vi "Constructor.vi"(10 "Beverage":refnum<class "Beverage.lvclass">, 11 "Milk in":refnum<class "Milk.lvclass">) -> (3 "Milk out":refnum<class "Milk.lvclass">)   [LabVIEW 2011, in "Milk.lvclass"]
uses:
  Milk.lvclass
  Beverage/Beverage.lvclass
  Milk.lvclass/Milk.ctl
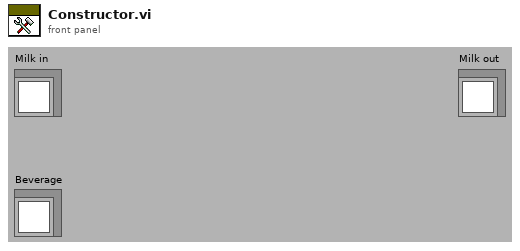
[diagram p1: front panel]
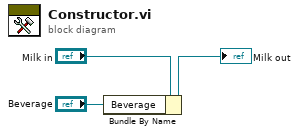
[diagram p0: block diagram]
diagram:
  n1 = Bundle By Name(cluster="Milk in", "Beverage"="Beverage") -> (→"Milk out":refnum<class "Milk.lvclass">)
